vi "get_skip_control_flag.vi"(8 "error in (no error)":errorcluster, 11 "ScanModeMG091111IntrinsicImaging in":refnum<class "ImagingModeMG091111IntrinsicImaging.lvclass">) -> (0 "error out":errorcluster, 2 "skip control?":bool, 3 "ScanModeMG091111IntrinsicImaging out":refnum<class "ImagingModeMG091111IntrinsicImaging.lvclass">)   [LabVIEW 2010, in "ImagingModeMG091111IntrinsicImaging.lvclass"]
uses:
  ImagingModeMG091111IntrinsicImaging.lvclass
  ImagingModeMG091111IntrinsicImaging.lvclass/ImagingModeMG091111IntrinsicImaging.ctl
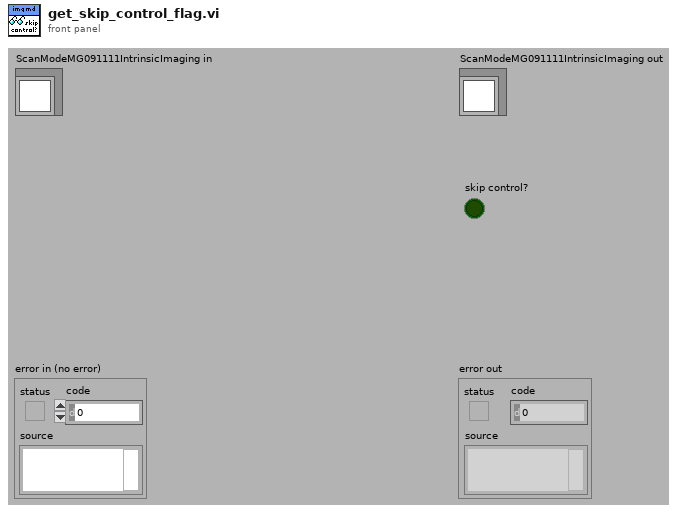
[diagram p1: front panel]
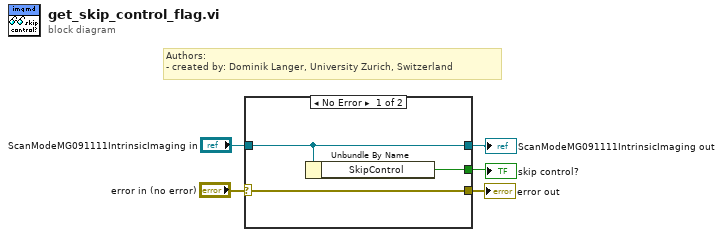
[diagram p0: block diagram]
diagram:
  # "Authors: \n- created by: Dominik Langer, University Zurich, Switzerland"
  n1 = case shown="No Error" "error in (no error)" {
    selector: "error in (no error)" -> [w8 w10]
    tunnel: [w8 w10] -> w4
    tunnel: [w7 w9] -> w2
    tunnel: "ScanModeMG091111IntrinsicImaging in" -> [w7 w9]
    tunnel: [w6 _] -> w1
    frame No Error {
      n2 = Unbundle By Name(w7) -> ("SkipControl"=w6:bool)
    }
    frame Error {
    }
  }
  "error out" <- w4
  "ScanModeMG091111IntrinsicImaging out" <- w2
  "skip control?" <- w1
